vi "Info.vi"(8 "ExitSendCmd":bool, 9 "Location":enum16{"CUMC", "SERI", "VMR", "Aline", "HSS"}(ring)=enum."HSS", 10 "base path":path, 11 "Patient Info In":T1={"Eye Selector"=enum."Right", "Plane"=12, "First Name"="", "Last Name"="", "Notes"="", "Patient ID"="", "Scan Location"=enum."Radio Selection 1"} {"Plane" min=1 max=12 step=1 scale=0.0..12.0}) -> (0 "NewCase?":bool, 1 "FileName":string, 3 "Patient Info Out":T1={"Eye Selector"=enum."Right", "Plane"=1, "First Name"="", "Last Name"="", "Notes"="", "Patient ID"="", "Scan Location"=enum."Radio Selection 1"} {"Plane" min=1 max=12 step=1 scale=0.0..12.0})   [LabVIEW 2022 SP3]
uses:
  -RT_support/PatientInfoDef.ctl
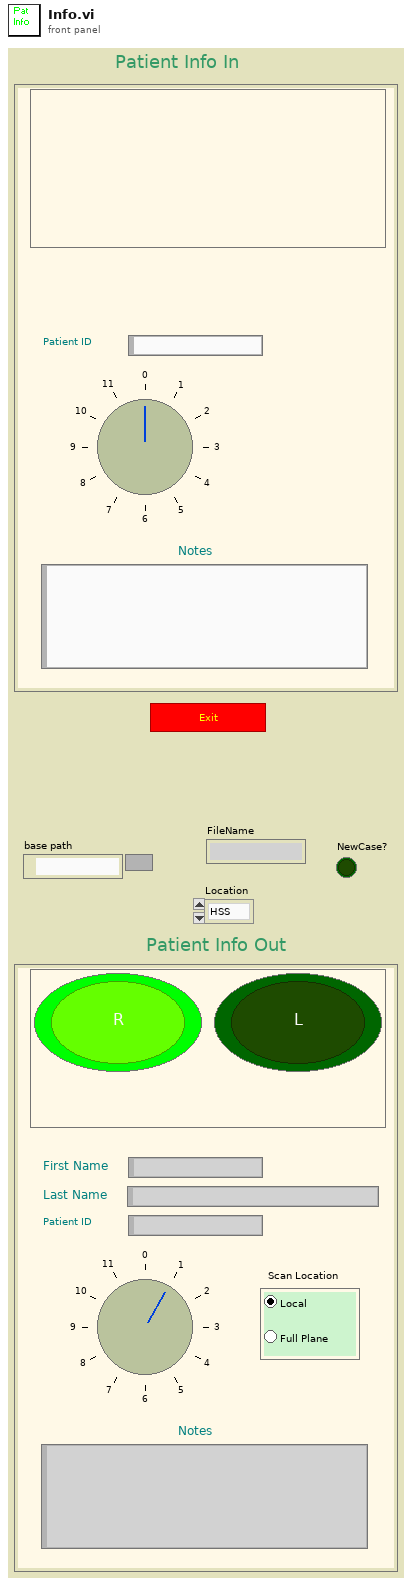
[diagram p1: front panel]
types:
  T1 = typedef "PatientInfoDef.ctl" = cluster{"Eye Selector":enum32{"Left", "Right"}, "Plane":i8, "First Name":string, "Last Name":string, "Notes":string, "Patient ID":string, "Scan Location":enum32{"Radio Selection 1", "Radio Selection 2"}}
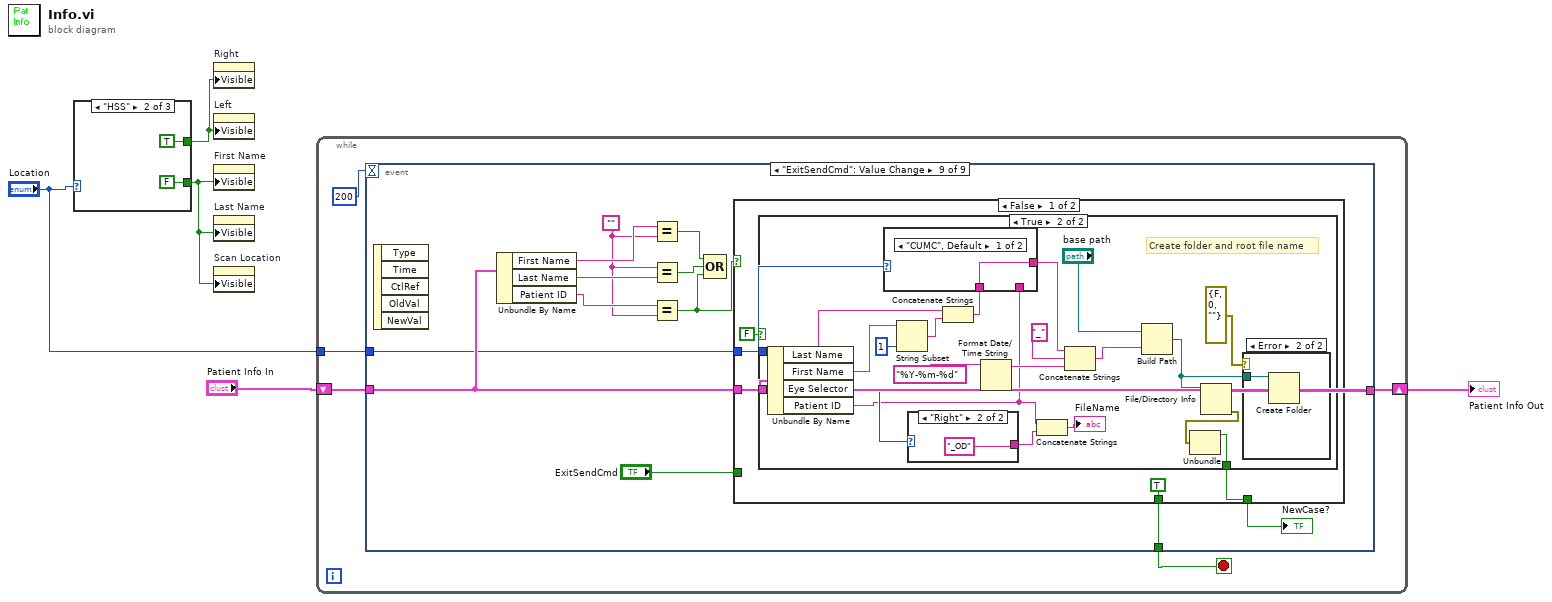
[diagram p0: block diagram]
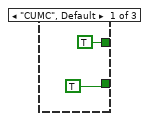
[diagram p2: hidden frame]
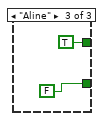
[diagram p3: hidden frame]
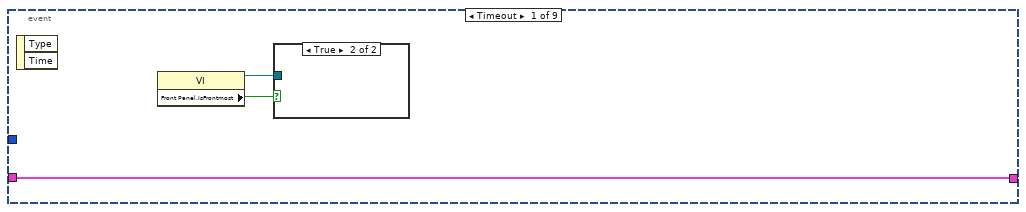
[diagram p4: hidden frame]
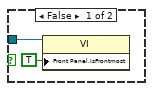
[diagram p5: hidden frame]
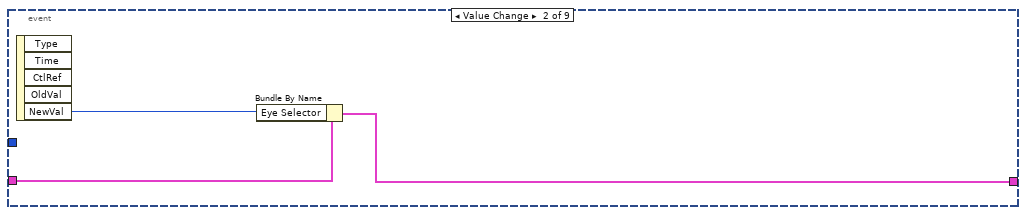
[diagram p6: hidden frame]
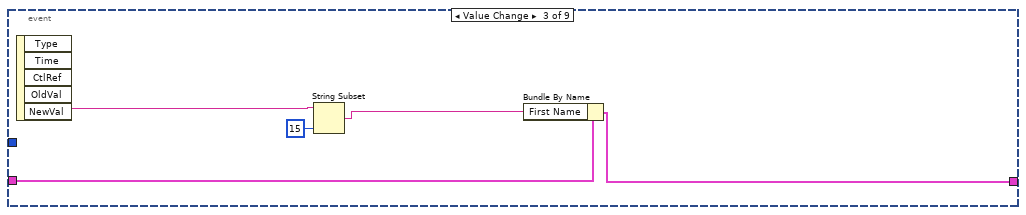
[diagram p7: hidden frame]
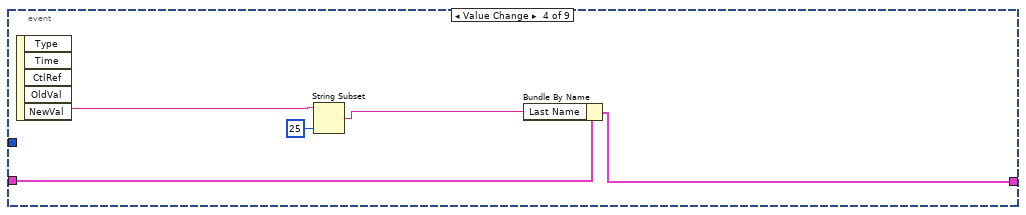
[diagram p8: hidden frame]
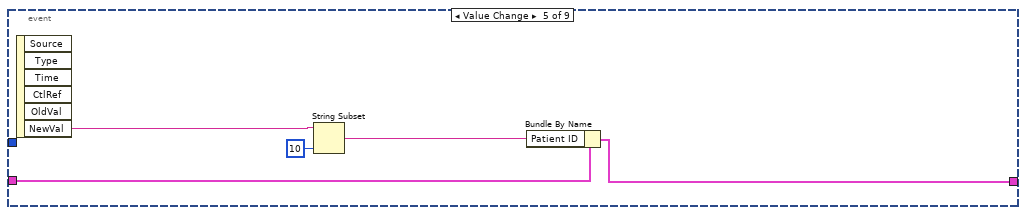
[diagram p9: hidden frame]
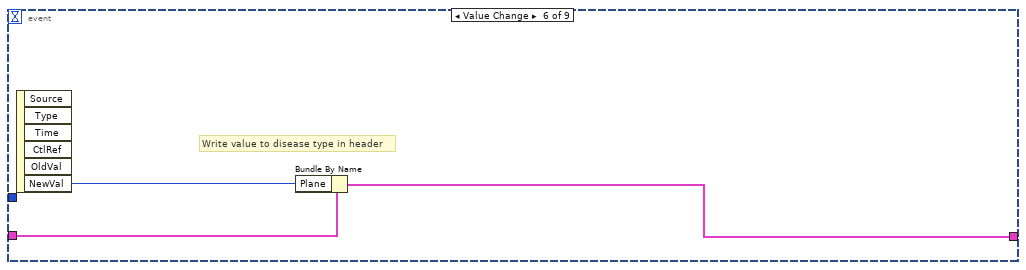
[diagram p10: hidden frame]
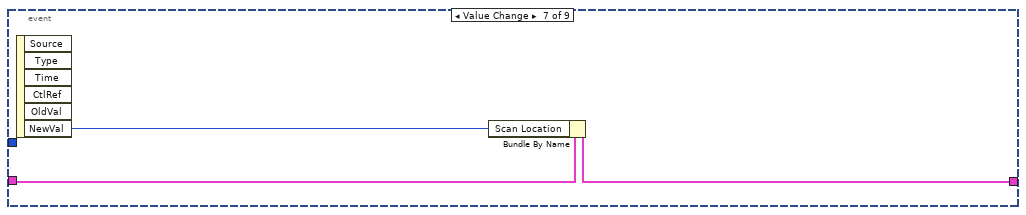
[diagram p11: hidden frame]
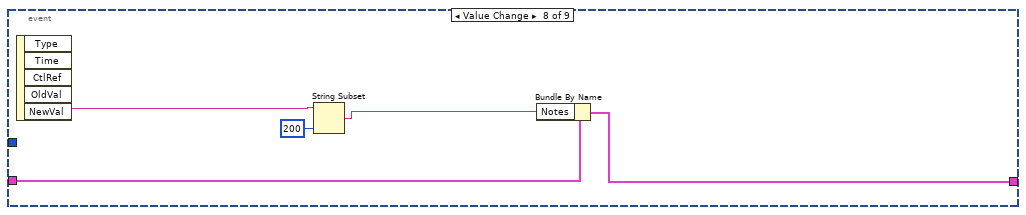
[diagram p12: hidden frame]
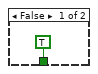
[diagram p13: hidden frame]
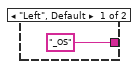
[diagram p16: hidden frame]
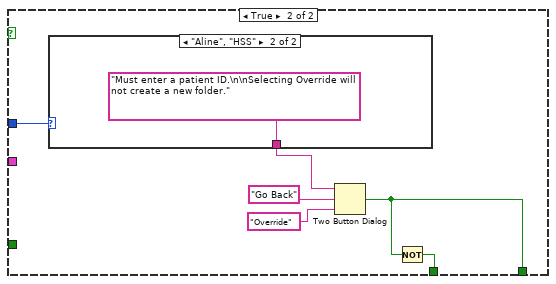
[diagram p17: hidden frame]
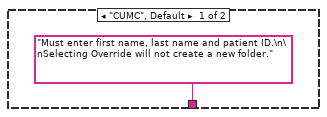
[diagram p18: hidden frame]
diagram:
  n1 = case shown="\"HSS\"" "Location" {
    tunnel: [TRUE ("Visible") FALSE ("Visible") FALSE ("Visible")] -> w3
    tunnel: [TRUE ("Visible") TRUE ("Visible") TRUE ("Visible")] -> w1
    frame "CUMC", Default {
    }
    frame "HSS" {
    }
    frame "Aline" {
    }
  }
  n2 = property on="Right" class="Bool (strict)"("Visible"=w1) -> ()  [unwired: 2 in, 2 out]
  n3 = property on="Left" class="Bool (strict)"("Visible"=w1) -> ()  [unwired: 2 in, 2 out]
  n4 = property on="First Name" class="Str"("Visible"=w3) -> ()  [unwired: 2 in, 2 out]
  n5 = property on="Last Name" class="Str"("Visible"=w3) -> ()  [unwired: 2 in, 2 out]
  n6 = property on="Scan Location" class="RadioBtnsControl (strict)"("Visible"=w3) -> ()  [unwired: 2 in, 2 out]
  n7 = while {
    shift-right: [w16] -> w5
    shift-left: "Patient Info In" -> [w15]
    tunnel: "Location" -> [w12]
    stop <- w13 stop-if-true
    n8 = event shown="[8] \"ExitSendCmd\": Value Change" {
      selector: _ -> [_ _ _ _ _ _ _ _ _]
      dyn-events: _ -> [_ _ _ _ _ _ _ _ _]
      timeout: 200 -> [_ _ _ _ _ _ _ _ _]
      tunnel: [w19 w23 w25 w30 w36 w41 w44 w46 w54] -> w16
      tunnel: w15 -> [w19 w24 w26 w31 w37 w42 w45 w47 w54]
      tunnel: [_ _ _ _ _ _ _ _ w59] -> w13
      tunnel: w12 -> [_ _ _ _ _ _ _ _ w51]
      event Timeout {
        n9 = event-data() -> ()  [unwired: 1 in, 2 out]
        n10 = property class="VI"() -> (reference out=w17:refnum<vi>, "Front Panel.IsFrontmost"=w18:bool)  [unwired: 2 in, 1 out]
        n11 = case shown="True" w18 {
          tunnel: w17 -> [w20 _]
          frame False {
            n12 = property class="VI"(reference=w20, "Front Panel.IsFrontmost"=TRUE ("Front Panel Window:Is Frontmost")) -> ()  [unwired: 1 in, 2 out]
          }
          frame True {
          }
        }
      }
      event Value Change {
        n13 = event-data() -> ("NewVal"=w22:enum32{"Left", "Right"})  [unwired: 1 in, 4 out]
        n14 = Bundle By Name(cluster=w24, "Eye Selector"=w22) -> (w23:T1)
      }
      event Value Change {
        n15 = event-data() -> ("NewVal"=w29:string)  [unwired: 1 in, 4 out]
        n16 = String Subset(string=w29, length (rest)=15 ("length (rest)")) -> (substring=w27:string)  [unwired: 1 in]
        n17 = Bundle By Name(cluster=w26, "First Name"=w27) -> (w25:T1)
      }
      event Value Change {
        n18 = event-data() -> ("NewVal"=w34:string)  [unwired: 1 in, 4 out]
        n19 = String Subset(string=w34, length (rest)=25 ("length (rest)")) -> (substring=w32:string)  [unwired: 1 in]
        n20 = Bundle By Name(cluster=w31, "Last Name"=w32) -> (w30:T1)
      }
      event Value Change {
        n21 = event-data() -> ("NewVal"=w35:string)  [unwired: 1 in, 5 out]
        n22 = String Subset(string=w35, length (rest)=10 ("length (rest)")) -> (substring=w38:string)  [unwired: 1 in]
        n23 = Bundle By Name(cluster=w37, "Patient ID"=w38) -> (w36:T1)
      }
      event Value Change {
        # "Write value to disease type in header"
        n24 = event-data() -> ("NewVal"=w40:i8)  [unwired: 1 in, 5 out]
        n25 = Bundle By Name(cluster=w42, "Plane"=w40) -> (w41:T1)
      }
      event Value Change {
        n26 = event-data() -> ("NewVal"=w43:enum32{"Radio Selection 1", "Radio Selection 2"})  [unwired: 1 in, 5 out]
        n27 = Bundle By Name(cluster=w45, "Scan Location"=w43) -> (w44:T1)
      }
      event Value Change {
        n28 = event-data() -> ("NewVal"=w50:string)  [unwired: 1 in, 4 out]
        n29 = String Subset(string=w50, length (rest)=200 ("length (rest)")) -> (substring=w48:string)  [unwired: 1 in]
        n30 = Bundle By Name(cluster=w47, "Notes"=w48) -> (w46:T1)
      }
      event "ExitSendCmd": Value Change {
        w56 = ""
        n31 = event-data() -> ()  [unwired: 1 in, 5 out]
        n32 = Unbundle By Name(w54) -> ("First Name"=w62:string, "Last Name"=w58:string, "Patient ID"=w57:string)
        n33 = Equal?(x=w62, y=w56) -> (x = y?=w61:bool)
        n34 = Equal?(x=w56, y=w58) -> (x = y?=w60:bool)
        n35 = Equal?(x=w57, y=w56) -> (x = y?=w52:bool)
        n36 = Compound Arithmetic op=OR(w61, w60, w52) -> ()  [unwired: 1 out]
        n37 = case shown="False" w52 {
          tunnel: [TRUE ("ExitSendCmd") w98] -> w59
          tunnel: "ExitSendCmd" -> [_ _]
          tunnel: w54 -> [w67 _]
          tunnel: [w65 w97] -> w53
          tunnel: w51 -> [w64 w95]
          frame False {
            n38 = case shown="True" FALSE {
              tunnel: w67 -> [_ w88]
              tunnel: [TRUE ("status") w74] -> w65
              tunnel: w64 -> [_ w73]
              frame False {
              }
              frame True {
                # "Create folder and root file name"
                n39 = Unbundle By Name(w88) -> ("Last Name"=w84:string, "First Name"=w86:string, "Eye Selector"=w87:enum32{"Left", "Right"}, "Patient ID"=w70:string)
                n40 = String Subset(string=w86, length (rest)=1 ("length (rest)")) -> (substring=w85:string)  [unwired: 1 in]
                n41 = case shown="\"Right\"" w87 {
                  tunnel: ["_OS" "_OD"] -> w81
                  frame "Left", Default {
                  }
                  frame "Right" {
                  }
                }
                n42 = Concatenate Strings(w84, w85) -> (w72:string)
                n43 = case shown="\"CUMC\", Default" w73 {
                  tunnel: [w90 w91] -> w71
                  tunnel: w72 -> [w90 _]
                  tunnel: w70 -> [_ w91]
                  frame "CUMC", Default {
                  }
                  frame "Aline" {
                  }
                }
                n44 = Format Date/Time String(time format string (%c)="%Y-%m-%d") -> (date/time string=w82:string)  [unwired: 2 in]
                n45 = Concatenate Strings(w70, w81) -> (→"FileName":string)
                n46 = Concatenate Strings(w71, "_", w82) -> (w76:string)
                n47 = Build Path(base path="base path", name or relative path=w76) -> (appended path=w78:path)
                n48 = File/Directory Info(path=w78) -> (error out=w75:errorcluster)  [unwired: 1 in, 6 out]
                n49 = Unbundle(w75) -> ("status"=w74:bool)  [unwired: 2 out]
                n50 = case shown="Error" errorcluster {"status"=FALSE, "code"=0, "source"=""} ("error IO") {
                  tunnel: w78 -> [_ w92]
                  frame No Error {
                  }
                  frame Error {
                    n51 = Create Folder(path (use dialog)=w92) -> ()  [unwired: 2 in, 3 out]
                  }
                }
              }
            }
          }
          frame True {
            n52 = case shown="\"Aline\", \"HSS\"" w95 {
              tunnel: ["Must enter first name, last name and patient ID.\n\nSelecting Override will not create a new folder." ("message") "Must enter a patient ID.\n\nSelecting Override will not create a new folder." ("message")] -> w96
              frame "CUMC", Default {
              }
              frame "Aline", "HSS" {
              }
            }
            n53 = Two Button Dialog(message=w96, 1:"Override" ("T button name (\"OK\")"), 2:"Go Back" ("F button name (\"Cancel\")")) -> (T button?=w97:bool)
            n54 = Not(x=w97) -> (.not. x?=w98:bool)
          }
        }
        "NewCase?" <- w53
      }
    }
  }
  "Patient Info Out" <- w5
